vi "GlobalFear.vi"() -> ()   [LabVIEW 2010]
panel:
  out "HR":dbl
  out "Stimulus":dbl
  out "Parameter Names":string[](array[string])
  in  "Parameter Values":T1
  out "Sound":dbl
  out "Shock":dbl
  out "Iteration":dbl
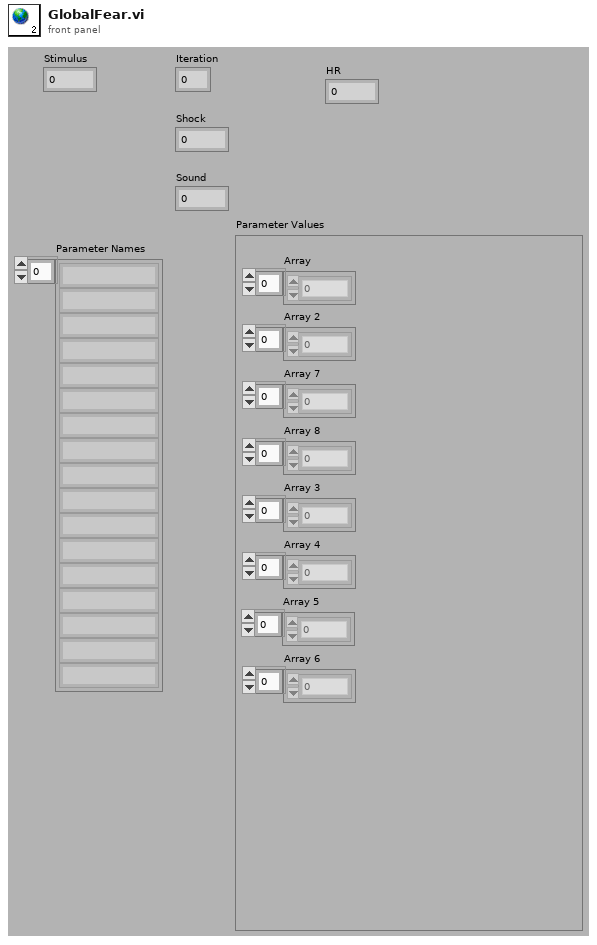
[diagram p1: front panel]
types:
  T1 = cluster{"Array":dbl[], "Array 2":dbl[], "Array 3":dbl[], "Array 4":dbl[], "Array 5":dbl[], "Array 6":dbl[], "Array 7":dbl[], "Array 8":dbl[]}
diagram:
